vi "AbortAll.vi"   [LabVIEW 2022 SP3]
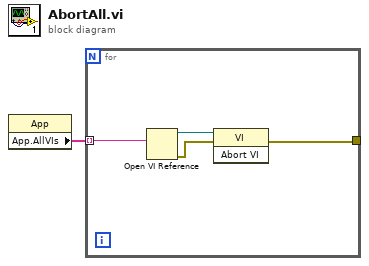
[diagram p0: block diagram]
diagram:
  n1 = property class="App"() -> ("App.AllVIs"=w1:string[])  [unwired: 2 in, 2 out]
  n2 = for {
    tunnel: w1 -> [w5] mode=indexing
    tunnel: [w2] -> _
    n3 = Open VI Reference(vi path=w5) -> (vi reference=w4:refnum<vi>, error out=w3:errorcluster)  [unwired: 5 in]
    n4 = invoke class="VI" method="Abort VI"(reference=w4, error in=w3) -> (error out=w2:errorcluster)  [unwired: 1 in, 2 out]
  }
